vi "subCreatePreBuiltLibrariesProjectItems.vi"(8 "error in":errorcluster, 11 "Lib definition strings":string[](array[string])) -> (0 "error out":errorcluster, 3 "Pre-built libraries":refnum<class "ProjectItem.lvclass">[](array[class]))   [LabVIEW 2019, in "SolutionBuilder.lvlib" / "SolutionBuilder.lvclass"]
uses:
  SolutionBuilder.lvclass
  ProjectItem/ProjectItem.lvclass
  ProjectItem/ProjectItem.lvclass/ProjectItem.ctl
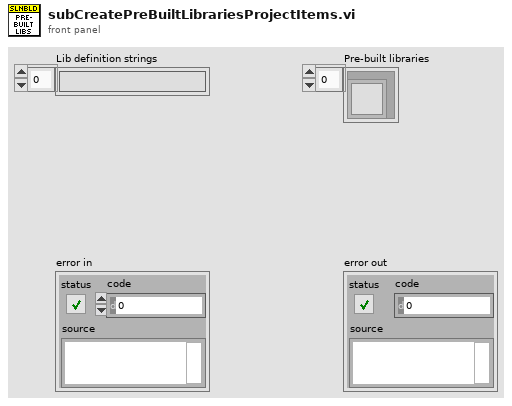
[diagram p1: front panel]
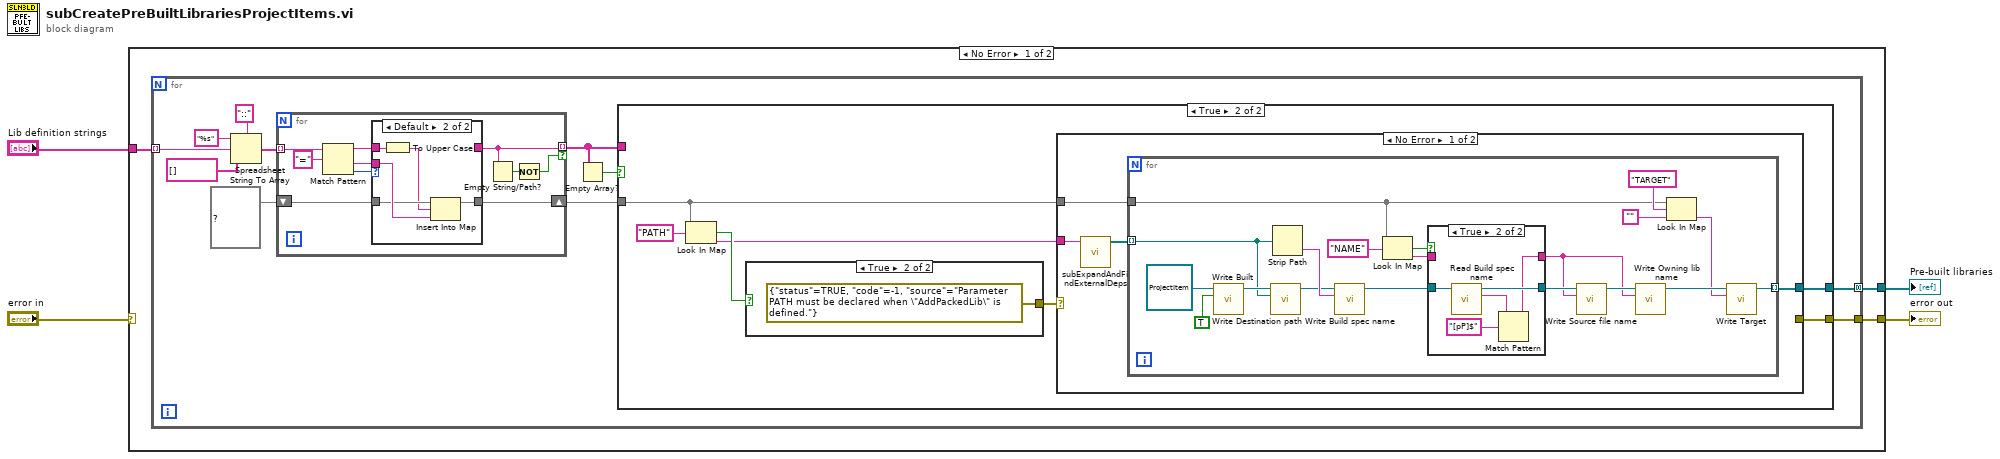
[diagram p0: block diagram]
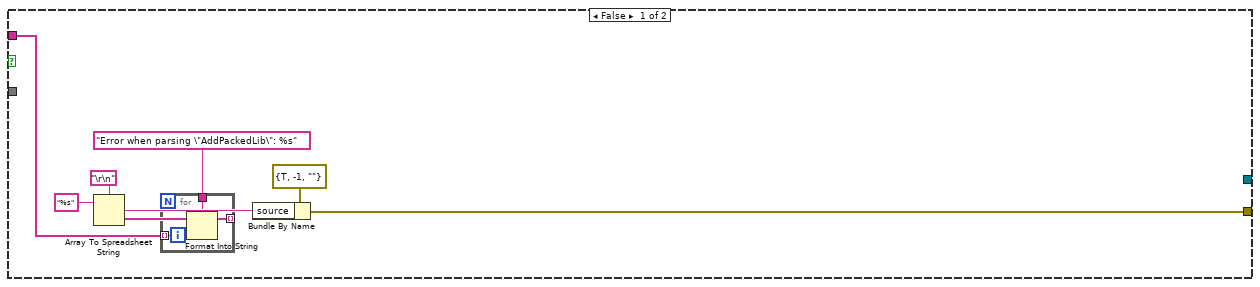
[diagram p2: hidden frame]
diagram:
  n1 = case shown="No Error" "error in" {
    selector: "error in" -> [_ w86]
    tunnel: "Lib definition strings" -> [w7 _]
    tunnel: [w6 w86] -> w2
    tunnel: [w5 _] -> w1
    frame No Error {
      n2 = for {
        tunnel: w7 -> [w15] mode=indexing
        tunnel: [w9] -> w5 mode=concatenating
        tunnel: [w8] -> w6
        n3 = Spreadsheet String To Array(delimiter (Tab)="::" ("regular expression"), format string="%s", spreadsheet string=w15, array type (2D Dbl)=string[] []) -> (array=w14:string[])
        n4 = for {
          tunnel: w14 -> [w77] mode=indexing
          shift-right: [w74] -> w12
          shift-left: map{string, string} {} ("map out") -> [w73]
          tunnel: [w71] -> w10 mode=indexing if=w69
          n5 = Match Pattern(string=w77, regular expression="=") -> (before substring=w76:string, after substring=w75:string, offset past match=w72:i32)  [unwired: 1 in, 1 out]
          n6 = case shown="Default" w72 {
            tunnel: w76 -> [w79 w85]
            tunnel: w75 -> [_ w84]
            tunnel: [w80 w83] -> w74
            tunnel: w73 -> [w80 w82]
            tunnel: [w79 _] -> w71
            frame -1 {
            }
            frame Default {
              n7 = To Upper Case(1:w85) -> (0:w81:string)
              n8 = Insert Into Map(map in=w82, key=w81, value=w84) -> (map out=w83:map{string, string})  [unwired: 2 out]
            }
          }
          n9 = Empty String/Path?(string/path=w71) -> (empty?=w70:bool)
          n10 = Not(x=w70) -> (.not. x?=w69:bool)
        }
        n11 = Empty Array?(array=w10) -> (empty?=w11:bool)
        n12 = case shown="True" w11 {
          tunnel: w12 -> [_ w34]
          tunnel: w10 -> [w20 _]
          tunnel: [_ w32] -> w9
          tunnel: [w19 w31] -> w8
          frame False {
            n13 = for {
              tunnel: w20 -> [w29] mode=indexing
              tunnel: [w28] -> w23 mode=indexing
              tunnel: "Error when parsing \"AddPackedLib\": %s" ("format string") -> [w27]
              n14 = Format Into String(format string=w27, w29) -> (resulting string=w28:string)  [unwired: 2 in, 1 out]
            }
            n15 = Array To Spreadsheet String(delimiter (Tab)="\r\n", array=w23, 3:"%s" ("format string")) -> (spreadsheet string=w24:string)
            n16 = Bundle By Name(cluster=errorcluster {"status"=TRUE, "code"=-1, "source"=""} ("error out"), "source"=w24) -> (w19:errorcluster)
          }
          frame True {
            n17 = Look In Map(map=w34, key="PATH" ("format string")) -> (key not found?=w36:bool, value=w30:string)  [unwired: 1 in]
            n18 = case shown="True" w36 {
              tunnel: [_ errorcluster {"status"=TRUE, "code"=-1, "source"="Parameter PATH must be declared when \"AddPackedLib\" is defined."} ("error out")] -> w33
              frame False {
              }
              frame True {
              }
            }
            n19 = case shown="No Error" w33 {
              selector: w33 -> [_ w67]
              tunnel: w34 -> [w40 _]
              tunnel: [w38 _] -> w32
              tunnel: [_ w67] -> w31
              tunnel: w30 -> [w37 _]
              frame No Error {
                n20 = call "subExpandAndFindExternalDeps.vi"("PATH in"=w37) -> ("Expanded deps"=w39:path[])  [unwired: 10 in]
                n21 = for {
                  tunnel: w40 -> [w52]
                  tunnel: [w49] -> w38 mode=indexing
                  tunnel: w39 -> [w42] mode=indexing
                  n22 = call "Write Built.vi"("Built"=TRUE, "ProjectItem in"=refnum<class "ProjectItem.lvclass"> refnum ("SolutionBuilder.lvlib:ProjectItem.lvclass")) -> ("ProjectItem out"=w48:refnum<class "ProjectItem.lvclass">)  [unwired: 9 in]
                  n23 = call "Write Destination path.vi"("Destination path"=w42, "ProjectItem in"=w48) -> ("ProjectItem out"=w46:refnum<class "ProjectItem.lvclass">)  [unwired: 9 in]
                  n24 = Strip Path(path=w42) -> (name=w47:string)  [unwired: 1 out]
                  n25 = call "Write Build spec name.vi"("Build spec name"=w47, "ProjectItem in"=w46) -> ("ProjectItem out"=w43:refnum<class "ProjectItem.lvclass">)  [unwired: 9 in]
                  n26 = Look In Map(map=w52, key="NAME" ("format string")) -> (key not found?=w57:bool, value=w59:string)  [unwired: 1 in]
                  n27 = case shown="True" w57 {
                    tunnel: w59 -> [w61 _]
                    tunnel: [w60 w63] -> w55
                    tunnel: w43 -> [w60 w66]
                    tunnel: [w61 w62] -> w54
                    frame False {
                    }
                    frame True {
                      n28 = call "Read Build spec name.vi"("ProjectItem in"=w66) -> ("Build spec name"=w64:string, "ProjectItem out"=w63:refnum<class "ProjectItem.lvclass">)  [unwired: 9 in]
                      n29 = Match Pattern(string=w64, regular expression="[pP]$") -> (before substring=w62:string)  [unwired: 1 in, 3 out]
                    }
                  }
                  n30 = call "Write Source file name.vi"("Source file name"=w54, "ProjectItem in"=w55) -> ("ProjectItem out"=w56:refnum<class "ProjectItem.lvclass">)  [unwired: 9 in]
                  n31 = call "Write Owning lib name.vi"("Owning lib name"=w54, "ProjectItem in"=w56) -> ("ProjectItem out"=w51:refnum<class "ProjectItem.lvclass">)  [unwired: 9 in]
                  n32 = Look In Map(map=w52, key="TARGET" ("format string"), default value="") -> (value=w50:string)  [unwired: 1 out]
                  n33 = call "Write Target.vi"("Target"=w50, "ProjectItem in"=w51) -> ("ProjectItem out"=w49:refnum<class "ProjectItem.lvclass">)  [unwired: 9 in]
                }
              }
              frame Error {
              }
            }
          }
        }
      }
    }
    frame Error {
    }
  }
  "error out" <- w2
  "Pre-built libraries" <- w1
